vi "GlueRepeatedLinePattern.vi"(2 "Controller In":refnum<k24>, 3 "Dry Run":bool, 4 "Stereo Angle [mrad]":dbl=-26.0 format="%#_13g", 5 "Module Number":i32=7, 6 "Calibration Directory":path) -> (0 ".NET Refnum out":refnum<k24>)   [LabVIEW 2016]
uses:
  <vilib>/LabVIEW Interface for Arduino/Type Defs/Arduino Resource.ctl
  <vilib>/LabVIEW Interface for Arduino/Type Defs/Board Type.ctl
  C:/Users/Aerotech/Documents/BNLStaveAssembly-blueprint/Bin/Aerotech.A3200.dll
  BNLStaveAssembly-blueprint/Bin/Aerotech.A3200.dll
  <vilib>/LabVIEW Interface for Arduino/Type Defs/Pin Mode.ctl
  <vilib>/Utility/file.llb/Read Delimited Spreadsheet (DBL).vi
  <vilib>/LabVIEW Interface for Arduino/LabVIEW Interface for Arduino.lvlib
panel:
  out "Line Motion":T1
  out "N Lines":i32
  out "Lines Glued":i32
  out "Elapsed Time [s]":dbl format="%.2g"
  out "Finished":bool
  in  "Abort stage":bool
  in  "Pattern Indicator":enum32{"Glue Pattern"}(tab)
  out "Relative Line\nSeparations [mm]":dbl[][](array[numeric])=[[18.5, 7.25], [2.5, 3.5], [-3.5, 5.0], [2.5, 3.15], [2.5, 3.15], [2.5, 3.15], [2.5, 3.15], [2.5, 3.15], [2.5, 3.15], [2.5, 3.15], [2.5, 3.15], [2.5, 3.15], [2.5, 3.15], [2.5, 3.15], [3.75, 5.0], [2.5, 3.5]] format="%#_13g"
  out "Line Lengths [mm]":dbl[](array[numeric])=[65.0, 65.0, 73.5, 73.5, 73.5, 73.5, 73.5, 73.5, 73.5, 73.5, 73.5, 73.5, 73.5, 73.5, 65.0, 65.0] format="%#_13g"
  in  "Outputs Tab":enum32{"Running Positions"}(tab)
  out "Running Positions [mm]":dbl[][](array[numeric])
  in  "Times [s]":dbl[](array[numeric])
  out "Running Times [s]":dbl[](array[numeric])
  in  "Inputs Tab":T2(tab)
  out "Virtual Stave Map":path
  out "Stave Angle [rad]":dbl format="%#_13g"
  out "Total Angle [rad]":dbl
  in  "Pulse Length [ms]":dbl=125.0 format="%#_13g"
  out "Arduino Resource":T3={"VISA resource"="GlueCTRL", "Board Type"=enum."Uno", "Connection Type"=enum."USB / Serial", "Bytes Per Packet (15)"=15}
  in  "Digital I/O Pin":u8=7
  in  "Default Axis Speeds":T5={"X [mm/s]"=25.0, "Y [mm/s]"=25.0, "Z [mm/s]"=25.0}
  in  "Camera to Dispenser \nShift [mm]":dbl[](array[numeric])=[109.832, 5.121, 0.0]
  in  "Glue Pattern .csv File":path=path "C:/Users/Aerotech/Documents/BNL_ThermomechanicalStave/SchillaciGlue/GluePatterns/Pattern3-1-v4.txt"
  in  "Axial":bool
  in  "Motion Time per Line [s]":dbl=6.75 format="%#_13g"
  in  "Wait [ms]":dbl=500.0 format="%#_13g"
  in  "Positions [mm]":dbl[][](array[numeric])
  in  "Terminate":bool
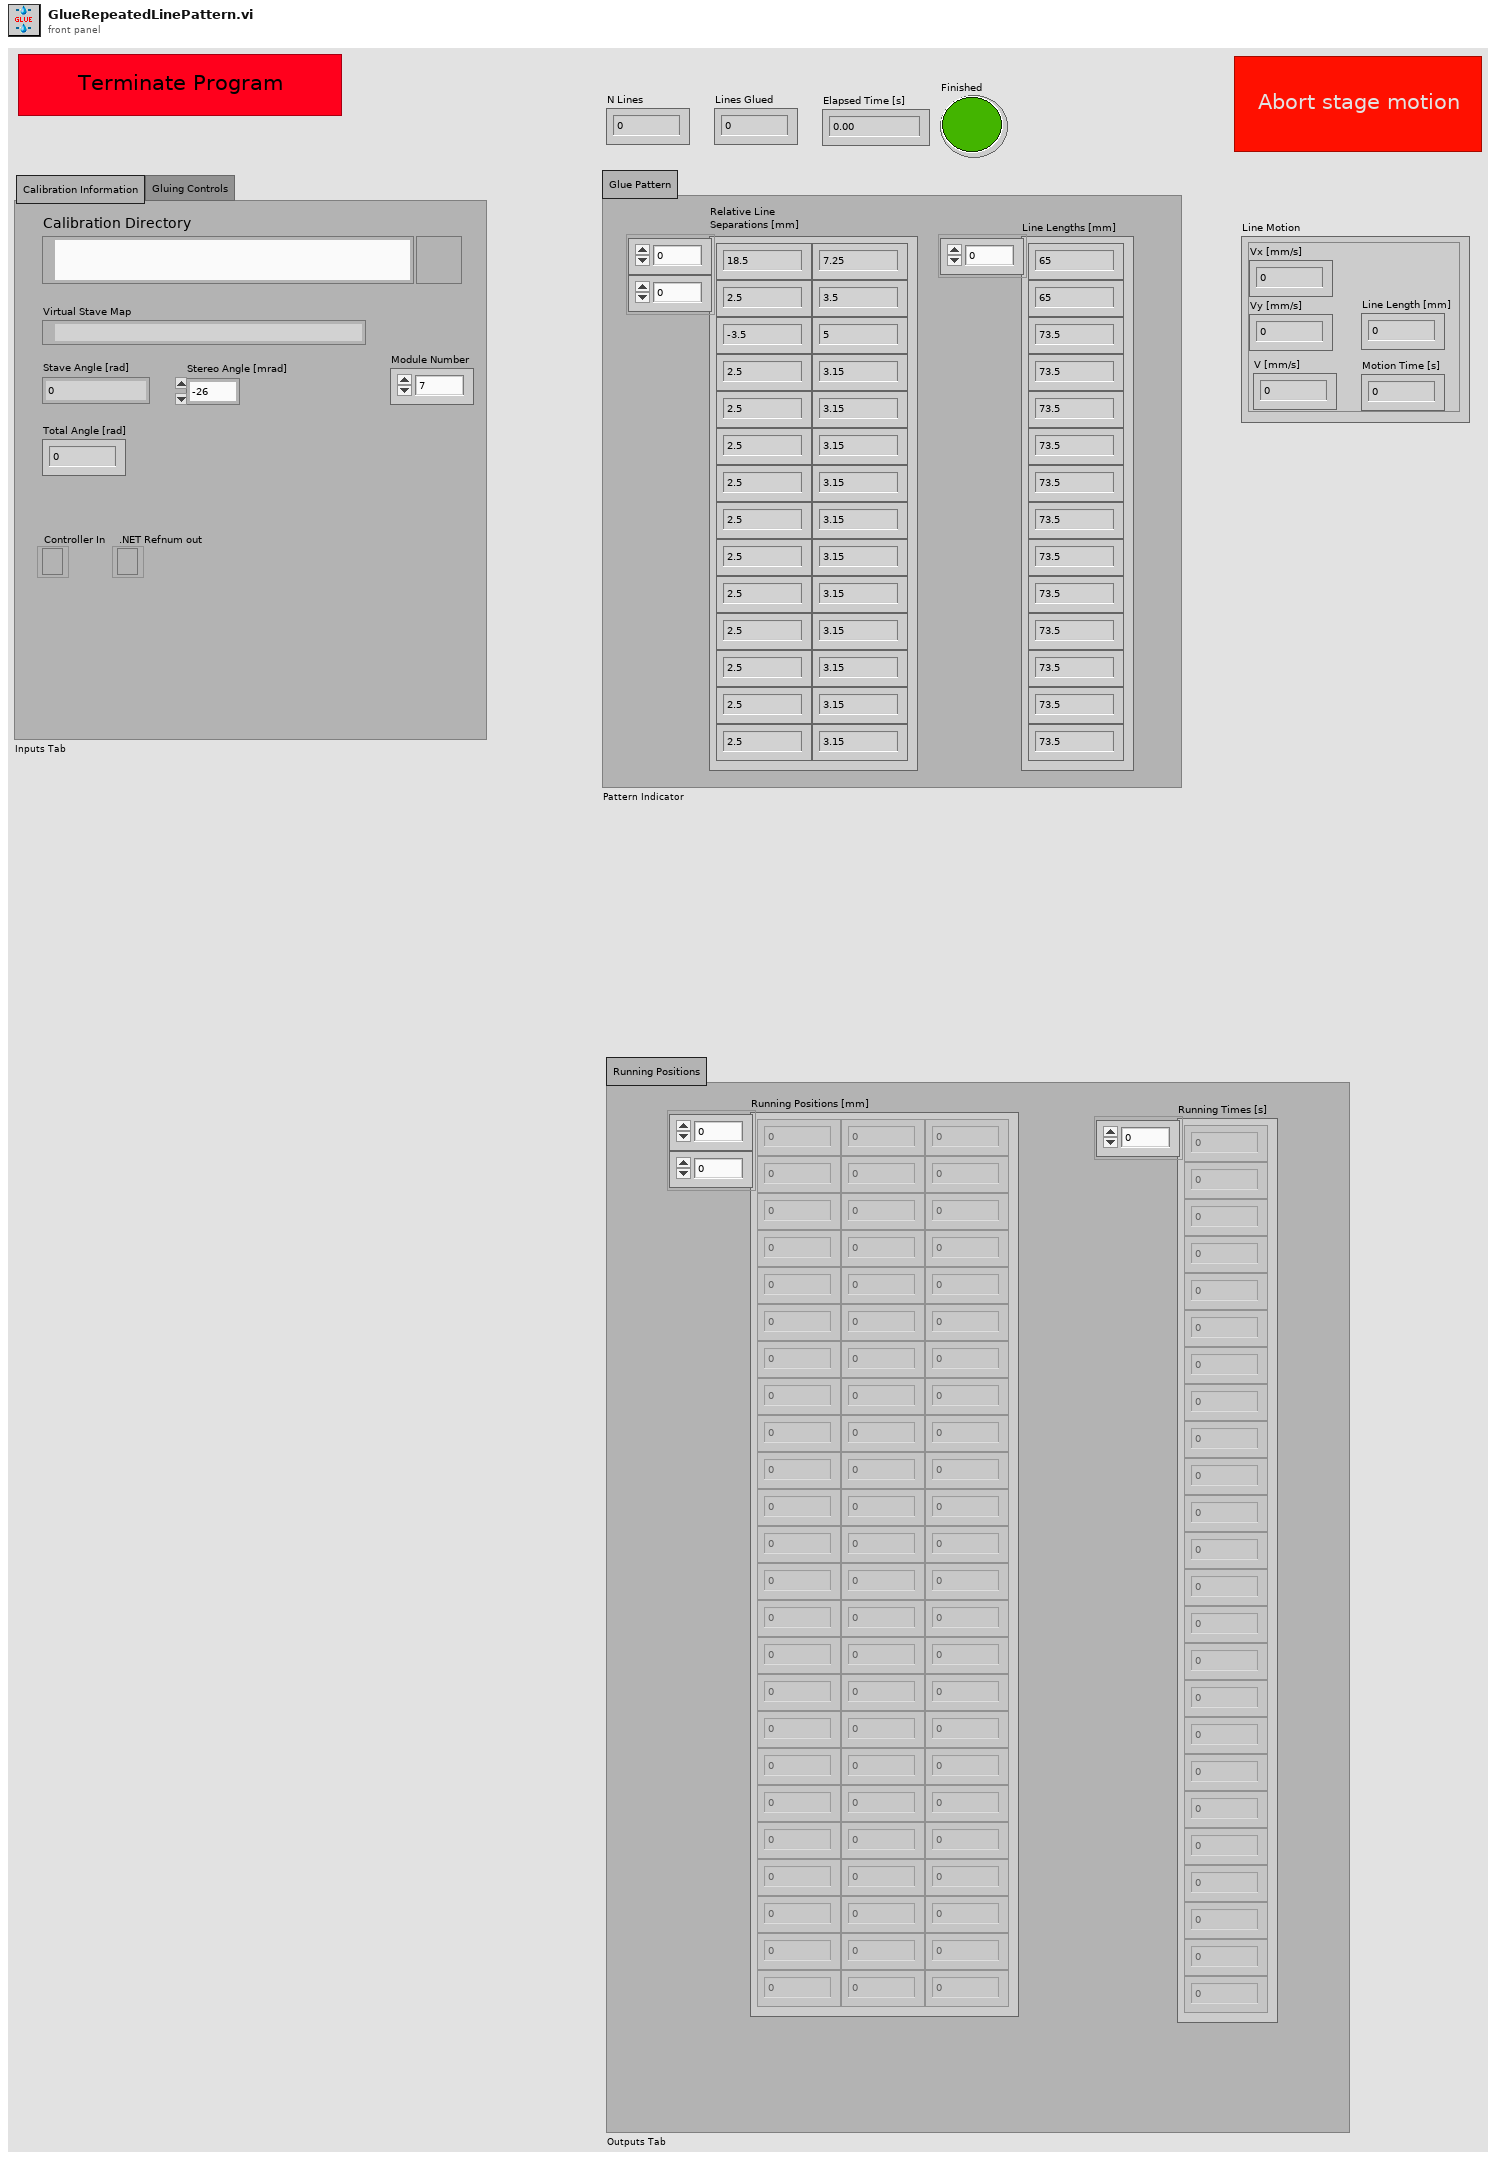
[diagram p1: front panel]
types:
  T1 = cluster{"Vx [mm/s]":dbl, "Vy [mm/s]":dbl, "Numeric Control":dbl, "Numeric Control":dbl, "Line Length [mm]":dbl}
  T2 = enum32{"Calibration Information", "Gluing Controls"}
  T3 = typedef "LabVIEW Interface for Arduino.lvlib/Arduino Resource.ctl" = cluster{"VISA resource":refnum<visa-resource-name>, "Board Type":T4, "Connection Type":enum8{"USB / Serial"}, "Bytes Per Packet (15)":u8}
  T4 = typedef "LabVIEW Interface for Arduino.lvlib/Board Type.ctl" = enum16{"Uno", "Dimuelanove w/Atmega 328", "Mega 2560"}
  T5 = cluster{"X [mm/s]":dbl, "Y [mm/s]":dbl, "Z [mm/s]":dbl}
  T6 = typedef "LabVIEW Interface for Arduino.lvlib/Pin Mode.ctl" = enum8{"Input", "Output"}
  T7 = cluster{"X [mm]":dbl, "Y [mm]":dbl, "Z [mm]":dbl}
  T8 = cluster{"Final X":dbl, "Final Y":dbl, "Final Z":dbl}
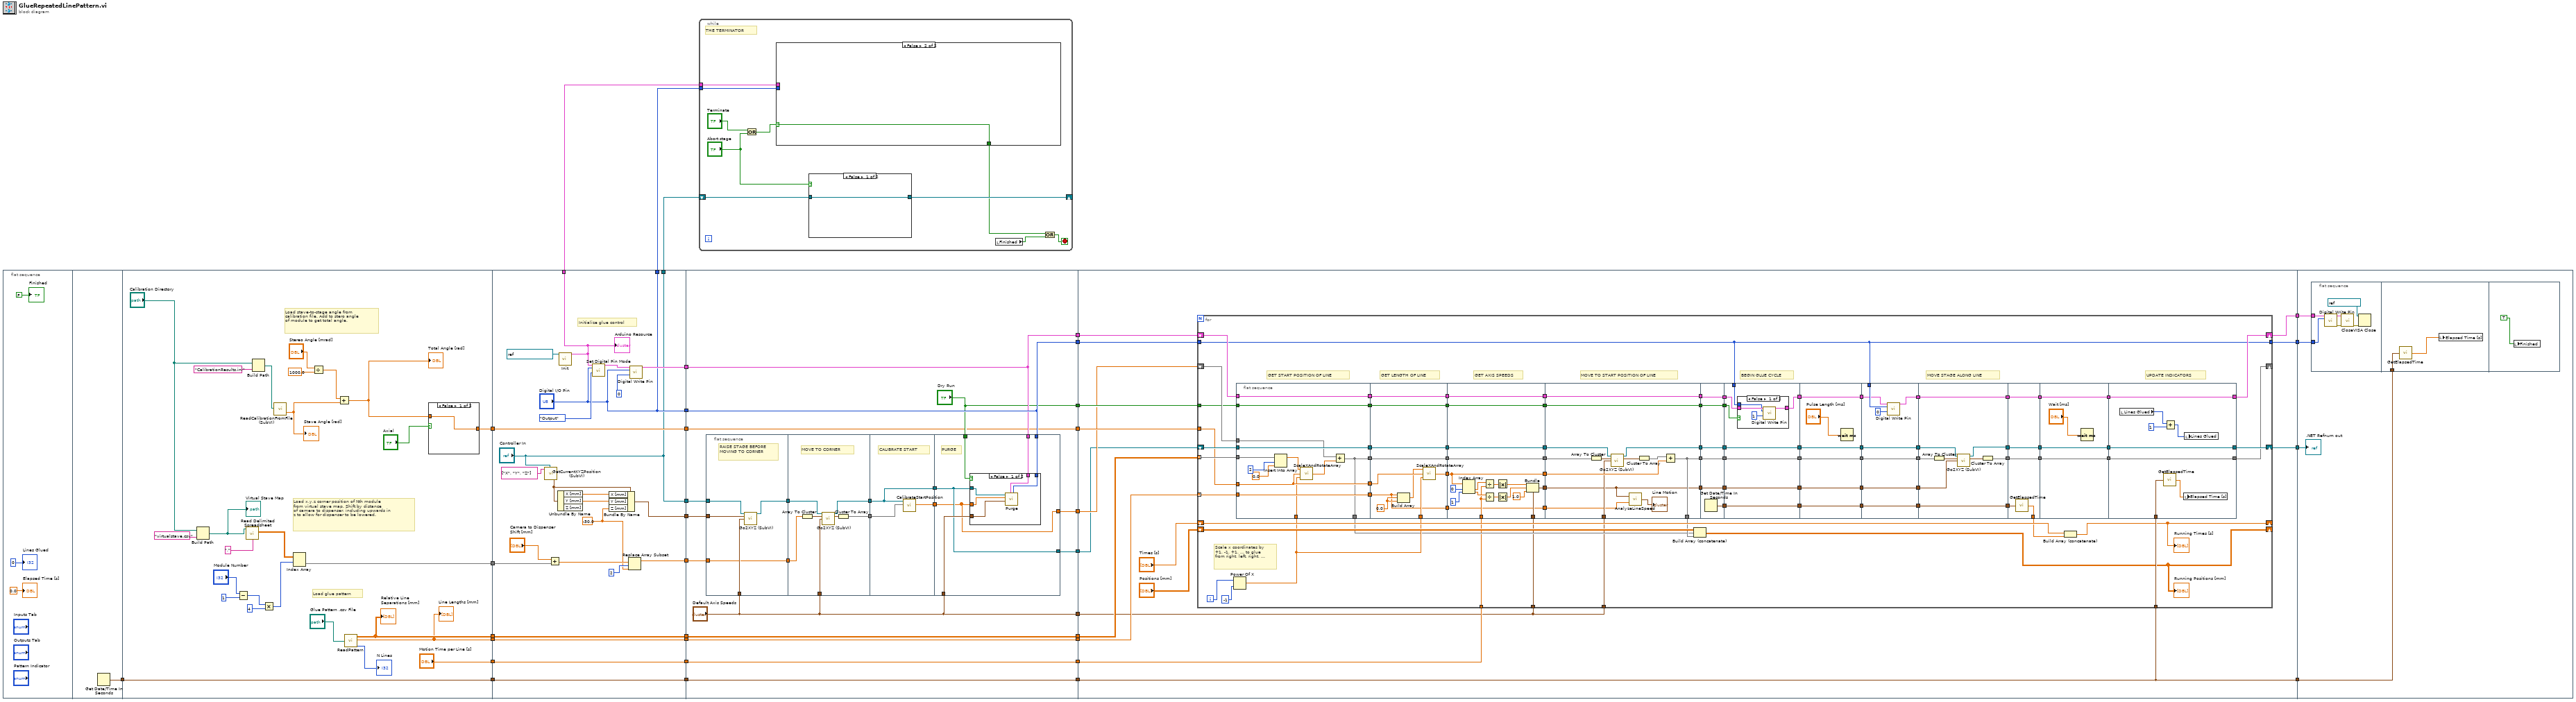
[diagram p0: block diagram]
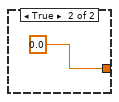
[diagram p2: hidden frame]
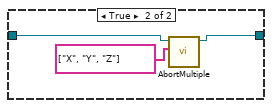
[diagram p5: hidden frame]
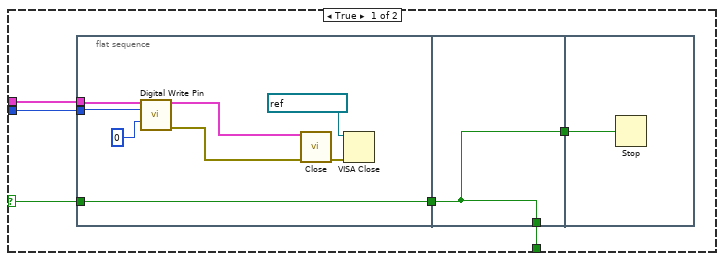
[diagram p6: hidden frame]
diagram:
  n1 = flat-sequence {
    tunnel: [w39] -> w21
    tunnel: w21 -> [w50]
    tunnel: [w50] -> w20
    tunnel: [w44] -> w16
    tunnel: [w47] -> w11
    tunnel: [w46] -> w10
    tunnel: [w42] -> w8
    tunnel: ["Motion Time per Line [s]"] -> w7
    tunnel: ["Controller In"] -> w35
    tunnel: [w87] -> w34
    tunnel: ["Digital I/O Pin"] -> w33
    tunnel: [w86] -> w27
    tunnel: ["Controller In"] -> w26
    tunnel: [w84] -> w23
    tunnel: w20 -> [w85]
    tunnel: [w85] -> w19
    tunnel: w16 -> [w84]
    tunnel: ["Digital I/O Pin"] -> w15
    tunnel: [w82] -> w12
    tunnel: w11 -> [w82]
    tunnel: w10 -> [w81]
    tunnel: [w81] -> w9
    tunnel: w8 -> [w74]
    tunnel: w7 -> [w80]
    tunnel: [w80] -> w6
    tunnel: [w68] -> w3
    tunnel: [w72] -> w2
    tunnel: w35 -> [w107]
    tunnel: w34 -> [w105]
    tunnel: w33 -> [w106]
    tunnel: [w106] -> w30
    tunnel: [w105] -> w29
    tunnel: [w104] -> w28
    tunnel: ["Dry Run"] -> w25
    tunnel: [w102] -> w24
    tunnel: w23 -> [w102]
    tunnel: [w101] -> w22
    tunnel: w19 -> [w100]
    tunnel: [w100] -> w18
    tunnel: [w99] -> w14
    tunnel: [w98] -> w13
    tunnel: w12 -> [w99]
    tunnel: w9 -> [w98]
    tunnel: w6 -> [w96]
    tunnel: [w96] -> w5
    tunnel: ["Default Axis Speeds"] -> w4
    tunnel: w3 -> [w93]
    tunnel: w2 -> [w92]
    tunnel: [w140] -> w32
    tunnel: [w152] -> w31
    tunnel: w30 -> [w151]
    tunnel: w29 -> [w150]
    tunnel: w28 -> [w146]
    tunnel: w25 -> [w149]
    tunnel: w24 -> [w148]
    tunnel: w22 -> [w147]
    tunnel: w18 -> [w145]
    tunnel: [w145] -> w17
    tunnel: w14 -> [w144]
    tunnel: w13 -> [w143]
    tunnel: w5 -> [w141]
    tunnel: w4 -> [w139]
    tunnel: [w138] -> w1
    tunnel: w32 -> [w351]
    tunnel: w31 -> [w350]
    tunnel: w17 -> [w349]
    tunnel: w1 -> [w348]
    frame #0 {
      "Finished" <- FALSE ("Finished")
      "Elapsed Time [s]" <- 0.0 ("Elapsed Time [s]")
      "Lines Glued" <- 0 ("N Lines")
    }
    frame #1 {
      n2 = Get Date/Time In Seconds() -> (seconds since 1Jan1904=w39:timestamp)
    }
    frame #2 {
      # "Load glue pattern"
      # "Load x,y,z corner position of Nth module\nfrom virtual stave map. Shift by distance\nof camera to dispenser, including upwards in\nz to allow for dispenser to be lowered."
      # "Load stave-to-stage angle from\ncalibration file. Add to stero angle\nof module to get total angle."
      n3 = Build Path(base path="Calibration Directory", name or relative path="virtualstave.csv") -> (appended path=w59:path)
      "Virtual Stave Map" <- w59
      n4 = Subtract(x="Module Number", y=1) -> (x-y=w55:i32)
      n5 = call-poly <vilib>:"Read Delimited Spreadsheet.vi"("file path (dialog if empty)"=w59, "delimiter (\\t)"="," ("delimiter (\\t)")) -> ("all rows"=w52:dbl[][])  [unwired: 8 in, 5 out]
      n6 = Build Path(base path="Calibration Directory", name or relative path="CalibrationResults.ini") -> (appended path=w61:path)
      n7 = Multiply(x=w55, y=4) -> (x*y=w51:i32)
      n8 = call "ReadCalibrationFromFile (SubVI).vi"("Calibration file path"=w61) -> ("Angle"=w40:dbl)  [unwired: 12 in, 6 out]
      "Stave Angle [rad]" <- w40
      n9 = Index Array(array=w52, index (row)=w51) -> (element=w42:dbl[])  [unwired: 1 in]
      n10 = Divide(x="Stereo Angle [mrad]", y=1000.0) -> (x/y=w53:dbl)
      n11 = Add(x=w53, y=w40) -> (x+y=w43:dbl)
      "Total Angle [rad]" <- w43
      n12 = call "ReadPattern.vi"("file path (dialog if empty)"="Glue Pattern .csv File") -> ("Relative Line\nSeparations [mm]"=w47:dbl[][], "Line Lengths [mm]"=w46:dbl[], "N Lines"=→"N Lines":i32)  [unwired: 1 in]
      "Relative Line\nSeparations [mm]" <- w47
      "Line Lengths [mm]" <- w46
      n13 = case shown="False" "Axial" {
        tunnel: [w66 0.0] -> w44
        tunnel: w43 -> [w66 _]
        frame False {
        }
        frame True {
        }
      }
    }
    frame #3 {
      w69 = -30.0 ("Z [mm]")
      # "Initialize glue control"
      n14 = call "GetCurrentXYZPosition (SubVI).vi"(".NET Refnum in - Device"="Controller In", "Axes Names"=string[] ["X", "Y", "Z"]) -> ("Current stage position"=w77:T7)  [unwired: 4 in, 5 out]
      n15 = Add(x="Camera to Dispenser \nShift [mm]", y=w74) -> (x+y=w71:dbl[])
      n16 = Unbundle By Name(w77) -> ("X [mm]"=w76:dbl, "Y [mm]"=w75:dbl)  [unwired: 1 out]
      n17 = call <vilib>:"Init.vi"("VISA resource"=refnum<visa-resource-name> "GlueCTRL") -> ("Arduino Resource"=w86:T3)  [unwired: 17 in, 1 out]
      "Arduino Resource" <- w86
      n18 = call <vilib>:"Set Digital Pin Mode.vi"("Arduino Resource"=w86, "Digital I/O Pin"="Digital I/O Pin", "Pin Mode (Input)"=Pin_Mode."Output") -> ("Arduino Resource"=w89:T3)  [unwired: 11 in, 1 out]
      n19 = Bundle By Name(cluster=w77, "X [mm]"=w76, "Y [mm]"=w75, "Z [mm]"=w69) -> (w72:T7)
      n20 = Replace Array Subset(array=w71, new element=w69, index=2) -> (w68:dbl[])
      n21 = call <vilib>:"Digital Write Pin.vi"("Arduino Resource"=w89, "Digital I/O Pin (0)"="Digital I/O Pin", "Value (0)"=u8 0) -> ("Arduino Resource"=w87:T3)  [unwired: 11 in, 1 out]
    }
    frame #4 {
      n22 = flat-sequence {
        tunnel: w107 -> [w116]
        tunnel: [w115] -> w97
        tunnel: "Default Axis Speeds" -> [w114]
        tunnel: [w113] -> w94
        tunnel: w93 -> [w113]
        tunnel: w92 -> [w112]
        tunnel: [w120] -> w111
        tunnel: [w119] -> w110
        tunnel: w97 -> [w121]
        tunnel: "Default Axis Speeds" -> [w118]
        tunnel: w94 -> [w117]
        tunnel: w111 -> [w125]
        tunnel: w110 -> [w126]
        tunnel: [w125] -> w109
        tunnel: [w124] -> w108
        tunnel: w109 -> [w129]
        tunnel: w108 -> [w127]
        tunnel: "Default Axis Speeds" -> [w132]
        tunnel: w106 -> [w131]
        tunnel: w105 -> [w130]
        tunnel: [w129] -> w104
        tunnel: "Dry Run" -> [w128]
        tunnel: [w127] -> w101
        frame #0 {
          # "RAISE STAGE BEFORE\nMOVING TO CORNER"
          n23 = call "Go2XYZ (SubVI).vi"(".NET Refnum in"=w116, "Go to Coordinates"=w112, "Axis Speeds"=w114) -> (".NET Refnum out"=w115:refnum<k24>)  [unwired: 8 in, 4 out]
        }
        frame #1 {
          # "MOVE TO CORNER"
          n24 = Array To Cluster(array=w117) -> (cluster=w123:cluster{"[0]":dbl, "[1]":dbl, "[2]":dbl})
          n25 = call "Go2XYZ (SubVI).vi"(".NET Refnum in"=w121, "Go to Coordinates"=w123, "Axis Speeds"=w118) -> (".NET Refnum out"=w120:refnum<k24>, "Final Position"=w122:T8)  [unwired: 8 in, 3 out]
          n26 = Cluster To Array(cluster=w122) -> (array=w119:dbl[])
        }
        frame #2 {
          # "CALIBRATE START"
          n27 = call "CalibrateStartPosition.vi"("Start Position [mm]"=w126, ".NET Refnum In"=w125) -> ("Final Position [mm]"=w124:dbl[])  [unwired: 9 in]
        }
        frame #3 {
          # "PURGE"
          n28 = case shown="False" w128 {
            tunnel: w132 -> [w135 _]
            tunnel: w131 -> [w137 _]
            tunnel: w130 -> [w136 _]
            tunnel: w129 -> [w133 _]
            tunnel: w127 -> [w134 _]
            frame False {
              n29 = call "Purge.vi"("Digital I/O Pin"=w137, "Arduino Resource"=w136, "Axis Speeds"=w135, "Start Position [mm]"=w134, ".NET Refnum In"=w133) -> ()  [unwired: 7 in]
            }
            frame True {
            }
          }
        }
      }
    }
    frame #5 {
      n30 = for {
        tunnel: w144 -> [w189] mode=indexing
        tunnel: w143 -> [w187] mode=indexing
        shift-right: [w227] -> _
        shift-left: w147 -> [w190]
        shift-right: [w228] -> w138
        shift-left: w146 -> [w231]
        shift-right: [w232] -> w140
        shift-left: w150 -> [w230]
        shift-right: [w208] -> _
        shift-left: "Positions [mm]" -> [w229]
        tunnel: w151 -> [w207]
        tunnel: [w207] -> w152
        tunnel: w149 -> [w186]
        tunnel: w148 -> [w185]
        tunnel: w145 -> [w225]
        shift-right: [w209] -> _
        shift-left: "Times [s]" -> [w220]
        tunnel: w141 -> [w164]
        tunnel: w139 -> [w157]
        tunnel: w139 -> [w156]
        i -> [w226]
        # "GET AXIS SPEEDS"
        # "BEGIN GLUE CYCLE"
        # "GET LENGTH OF LINE"
        # "GET START POSITION OF LINE"
        # "UPDATE INDICATORS"
        # "MOVE STAGE ALONG LINE"
        # "MOVE TO START POSITION OF LINE"
        # "Scale x coordinates by\n+1, -1, +1, ... to glue\nfrom right, left, right, ..."
        n31 = Power Of X(1:-1 ("x"), 2:w226) -> (0:w183:dbl)
        n32 = flat-sequence {
          tunnel: w186 -> [w244]
          tunnel: w231 -> [w245]
          tunnel: w230 -> [w246]
          tunnel: [w246] -> w194
          tunnel: [w245] -> w193
          tunnel: [w244] -> w192
          tunnel: [w234] -> w191
          tunnel: w190 -> [w243]
          tunnel: w189 -> [w240]
          tunnel: [w237] -> w188
          tunnel: w187 -> [w237]
          tunnel: w185 -> [w236]
          tunnel: [w236] -> w184
          tunnel: w183 -> [w235]
          tunnel: [w234] -> w181
          tunnel: [w256] -> w180
          tunnel: [w255] -> w178
          tunnel: [w254] -> w176
          tunnel: [w253] -> w174
          tunnel: [w252] -> w172
          tunnel: w194 -> [w256]
          tunnel: w193 -> [w255]
          tunnel: w192 -> [w254]
          tunnel: w191 -> [w253]
          tunnel: w188 -> [w247]
          tunnel: w184 -> [w250]
          tunnel: w183 -> [w248]
          tunnel: [w247] -> w154
          tunnel: w180 -> [w274]
          tunnel: [w274] -> w179
          tunnel: w178 -> [w273]
          tunnel: [w273] -> w177
          tunnel: w176 -> [w272]
          tunnel: [w272] -> w175
          tunnel: w174 -> [w271]
          tunnel: [w271] -> w173
          tunnel: w172 -> [w269]
          tunnel: [w269] -> w171
          tunnel: w164 -> [w264]
          tunnel: [w263] -> w163
          tunnel: w156 -> [w258]
          tunnel: [w257] -> w155
          tunnel: w154 -> [w257]
          tunnel: [w288] -> w224
          tunnel: [w279] -> w223
          tunnel: [w282] -> w222
          tunnel: [w287] -> w221
          tunnel: w179 -> [w288]
          tunnel: w177 -> [w280]
          tunnel: w175 -> [w287]
          tunnel: w173 -> [w281]
          tunnel: w171 -> [w283]
          tunnel: [w282] -> w182
          tunnel: w163 -> [w275]
          tunnel: [w275] -> w160
          tunnel: w157 -> [w278]
          tunnel: w155 -> [w277]
          tunnel: w224 -> [w294]
          tunnel: [w294] -> w218
          tunnel: w223 -> [w293]
          tunnel: [w293] -> w217
          tunnel: w222 -> [w292]
          tunnel: [w292] -> w216
          tunnel: w221 -> [w291]
          tunnel: [w291] -> w215
          tunnel: [w290] -> w214
          tunnel: [w289] -> w161
          tunnel: w160 -> [w289]
          tunnel: w218 -> [w299]
          tunnel: w217 -> [w302]
          tunnel: [w302] -> w202
          tunnel: w216 -> [w301]
          tunnel: [w301] -> w200
          tunnel: w215 -> [w297]
          tunnel: w214 -> [w300]
          tunnel: [w300] -> w198
          tunnel: w207 -> [w296]
          tunnel: [w298] -> w196
          tunnel: [w295] -> w162
          tunnel: w161 -> [w295]
          tunnel: w202 -> [w313]
          tunnel: [w313] -> w201
          tunnel: w200 -> [w312]
          tunnel: [w312] -> w199
          tunnel: w198 -> [w311]
          tunnel: [w311] -> w197
          tunnel: w196 -> [w310]
          tunnel: [w310] -> w195
          tunnel: w162 -> [w308]
          tunnel: [w308] -> w158
          tunnel: w201 -> [w321]
          tunnel: [w321] -> w213
          tunnel: w199 -> [w320]
          tunnel: [w320] -> w212
          tunnel: w197 -> [w319]
          tunnel: [w319] -> w211
          tunnel: w195 -> [w316]
          tunnel: [w315] -> w210
          tunnel: w207 -> [w317]
          tunnel: [w314] -> w159
          tunnel: w158 -> [w314]
          tunnel: [w322] -> w206
          tunnel: w213 -> [w323]
          tunnel: w212 -> [w330]
          tunnel: [w329] -> w205
          tunnel: [w328] -> w204
          tunnel: w211 -> [w328]
          tunnel: w210 -> [w327]
          tunnel: [w327] -> w203
          tunnel: w159 -> [w326]
          tunnel: [w331] -> w170
          tunnel: w206 -> [w335]
          tunnel: [w335] -> w168
          tunnel: w205 -> [w334]
          tunnel: [w334] -> w166
          tunnel: w204 -> [w333]
          tunnel: [w332] -> w219
          tunnel: w203 -> [w331]
          tunnel: w170 -> [w339]
          tunnel: [w339] -> w169
          tunnel: w168 -> [w338]
          tunnel: [w338] -> w167
          tunnel: w166 -> [w337]
          tunnel: [w337] -> w165
          tunnel: [w347] -> w232
          tunnel: w169 -> [w347]
          tunnel: [w346] -> w228
          tunnel: w167 -> [w346]
          tunnel: [w345] -> w227
          tunnel: w165 -> [w345]
          tunnel: w225 -> [w341]
          frame #0 {
            n33 = Insert Into Array(array=w240, index=2, new element=0.0 ("new element/subarray")) -> (w239:dbl[])
            n34 = call "ScaleXAndRotateArray.vi"("Scale"=w235, "Angle"=w236, "X, Y, Z Input"=w239) -> ("c * X', Y', Z Output"=w238:dbl[])
            n35 = Add(x=w243, y=w238) -> (x+y=w234:dbl[])
          }
          frame #1 {
            w251 = 0.0 ("element")
            n36 = Build Array(w247, w251, w251) -> (w249:dbl[])
            n37 = call "ScaleXAndRotateArray.vi"("Scale"=w248, "Angle"=w250, "X, Y, Z Input"=w249) -> ("c * X', Y', Z Output"=w252:dbl[])
          }
          frame #2 {
            n38 = Index Array(array=w269, index #1=0 ("index"), index #2=1 ("index")) -> (element #1=w266:dbl, element #2=w265:dbl)
            n39 = Divide(x=w266, y=w264) -> (x/y=w262:dbl)
            n40 = Divide(x=w265, y=w264) -> (x/y=w261:dbl)
            n41 = Absolute Value(x=w262) -> (abs(x)=w260:dbl)
            n42 = Absolute Value(x=w261) -> (abs(x)=w259:dbl)
            n43 = Bundle(cluster=w258, "X [mm/s]"=w260, "Y [mm/s]"=w259, "Z [mm/s]"=1.0) -> (w263:T5)
          }
          frame #3 {
            n44 = Array To Cluster(array=w281) -> (cluster=w284:cluster{"[0]":dbl, "[1]":dbl, "[2]":dbl})
            n45 = call "Go2XYZ (SubVI).vi"(".NET Refnum in"=w280, "Go to Coordinates"=w284, "Axis Speeds"=w278) -> (".NET Refnum out"=w279:refnum<k24>, "Final Position"=w285:T8)  [unwired: 8 in, 3 out]
            n46 = call "AnalyzeLineSpeed.vi"("Line Length [mm]"=w277, "Line Speeds [mm/s]"=w275) -> ("Output"=→"Line Motion":T1)
            n47 = Cluster To Array(cluster=w285) -> (array=w286:dbl[])
            n48 = Add(x=w286, y=w283) -> (x+y=w282:dbl[])
          }
          frame #4 {
            n49 = Get Date/Time In Seconds() -> (seconds since 1Jan1904=w290:timestamp)
          }
          frame #5 {
            n50 = case shown="False" w297 {
              tunnel: [w306 w307] -> w298
              tunnel: w299 -> [w305 w307]
              tunnel: w296 -> [w303 _]
              frame False {
                n51 = call <vilib>:"Digital Write Pin.vi"("Arduino Resource"=w305, "Digital I/O Pin (0)"=w303, "Value (0)"=u8 1) -> ("Arduino Resource"=w306:T3)  [unwired: 11 in, 1 out]
              }
              frame True {
              }
            }
          }
          frame #6 {
            n52 = Wait (ms)(milliseconds to wait="Pulse Length [ms]") -> ()  [unwired: 1 out]
          }
          frame #7 {
            n53 = call <vilib>:"Digital Write Pin.vi"("Arduino Resource"=w316, "Digital I/O Pin (0)"=w317, "Value (0)"=u8 0) -> ("Arduino Resource"=w315:T3)  [unwired: 11 in, 1 out]
          }
          frame #8 {
            n54 = Array To Cluster(array=w330) -> (cluster=w324:cluster{"[0]":dbl, "[1]":dbl, "[2]":dbl})
            n55 = call "Go2XYZ (SubVI).vi"(".NET Refnum in"=w323, "Go to Coordinates"=w324, "Axis Speeds"=w326) -> (".NET Refnum out"=w322:refnum<k24>, "Final Position"=w325:T8)  [unwired: 8 in, 3 out]
            n56 = Cluster To Array(cluster=w325) -> (array=w329:dbl[])
          }
          frame #9 {
            n57 = call "GetElapsedTime.vi"("Start Time"=w333) -> ("Elapsed Time [s]"=w332:sgl)
          }
          frame #10 {
            n58 = Wait (ms)(milliseconds to wait="Wait [ms]") -> ()  [unwired: 1 out]
          }
          frame #11 {
            n59 = local read "Lines Glued"() -> (w343:i32)
            n60 = call "GetElapsedTime.vi"("Start Time"=w341) -> ("Elapsed Time [s]"=w340:sgl)
            n61 = Add(x=w343, y=1) -> (x+y=w344:i32)
            n62 = local write "Elapsed Time [s]"(w340) -> ()
            n63 = local write "Lines Glued"(w344) -> ()
          }
        }
        n64 = Build Array (concatenate)(w229, w181, w182) -> (w208:dbl[][])
        "Running Positions [mm]" <- w208
        n65 = Build Array (concatenate)(w220, w219) -> (w209:dbl[])
        "Running Times [s]" <- w209
      }
    }
    frame #6 {
      n66 = flat-sequence {
        tunnel: w351 -> [w353]
        tunnel: w350 -> [w352]
        tunnel: w349 -> [w358]
        frame #0 {
          n67 = call <vilib>:"Digital Write Pin.vi"("Arduino Resource"=w353, "Digital I/O Pin (0)"=w352) -> ("Arduino Resource"=w356:T3, "error out"=w355:errorcluster)  [unwired: 12 in]
          n68 = call <vilib>:"Close.vi"("Arduino Resource"=w356, "error in"=w355) -> ("error out"=w354:errorcluster)  [unwired: 13 in]
          n69 = VISA Close(VISA resource name=refnum<visa-resource-name> "GlueCTRL", error in (no error)=w354) -> ()  [unwired: 1 out]
        }
        frame #1 {
          n70 = call "GetElapsedTime.vi"("Start Time"=w358) -> ("Elapsed Time [s]"=w359:sgl)
          n71 = local write "Elapsed Time [s]"(w359) -> ()
        }
        frame #2 {
          n72 = local write "Finished"(TRUE ("stop? (T)")) -> ()
        }
      }
      ".NET Refnum out" <- w348
    }
  }
  n73 = while {
    tunnel: w27 -> [w370]
    shift-right: [w368] -> _
    shift-left: w26 -> [w369]
    tunnel: w15 -> [w362]
    stop <- w365 stop-if-true
    # "THE TERMINATOR"
    n74 = Or(x="Terminate", y="Abort stage") -> (x .or. y?=w364:bool)
    n75 = case shown="False" w364 {
      selector: w364 -> [w380 w391]
      tunnel: w370 -> [w378 _]
      tunnel: [w376 w391] -> w363
      tunnel: w362 -> [w375 _]
      frame True {
        n76 = flat-sequence {
          tunnel: [w386] -> w379
          tunnel: w375 -> [w382]
          tunnel: w378 -> [w384]
          tunnel: w380 -> [w386]
          tunnel: w379 -> [w389]
          tunnel: [w389] -> w377
          tunnel: [w389] -> w376
          tunnel: w377 -> [w390]
          frame #0 {
            n77 = call <vilib>:"Digital Write Pin.vi"("Arduino Resource"=w384, "Digital I/O Pin (0)"=w382, "Value (0)"=u8 0) -> ("Arduino Resource"=w385:T3, "error out"=w381:errorcluster)  [unwired: 11 in]
            n78 = call <vilib>:"Close.vi"("Arduino Resource"=w385, "error in"=w381) -> ("error out"=w387:errorcluster)  [unwired: 13 in]
            n79 = VISA Close(VISA resource name=refnum<visa-resource-name> "GlueCTRL", error in (no error)=w387) -> ()  [unwired: 1 out]
          }
          frame #1 {
          }
          frame #2 {
            n80 = Stop(stop? (T)=w390) -> ()
          }
        }
      }
      frame False {
      }
    }
    n81 = case shown="False" "Abort stage" {
      tunnel: w369 -> [w371 w373]
      tunnel: [w371 w372] -> w368
      frame False {
      }
      frame True {
        n82 = call "AbortMultiple.vi"("axis names"=string[] ["X", "Y", "Z"], "controller in"=w373) -> ("controller out"=w372:refnum<k24>)  [unwired: 8 in, 1 out]
      }
    }
    n83 = local read "Finished"() -> (w361:bool)
    n84 = Or(x=w363, y=w361) -> (x .or. y?=w365:bool)
  }
